vi "setUp.vi"(8 "error in (no error)":errorcluster, 11 "reference in":refnum<class "UnitTestIntClass.lvclass">) -> (0 "error out":errorcluster, 3 "reference in":refnum<class "UnitTestIntClass.lvclass">)   [LabVIEW 2011, in "UnitTestIntClass.lvclass"]
doc: "setUp runs prior to the test method during test execution. Use this method to initialize any object data required by your tests."
uses:
  UnitTestIntClass.lvclass
  UnitTestIntClass.lvclass/UnitTestIntClass.ctl
  IntClass/IntClass.lvclass
  <vilib>/addons/_JKI Toolkits/VI Tester/TestCase.llb/TestCase.lvclass
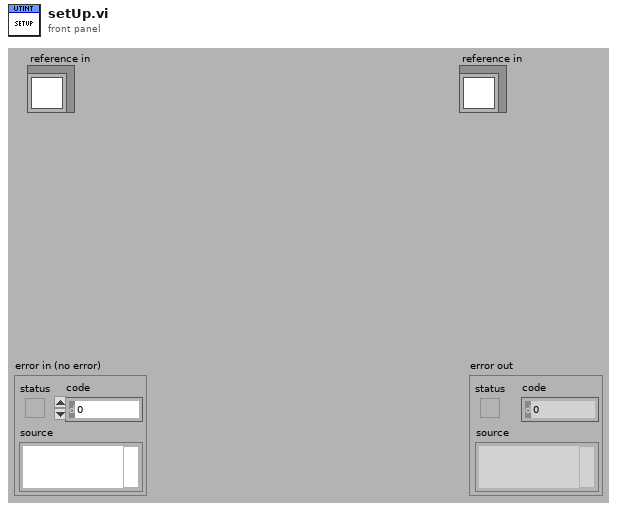
[diagram p1: front panel]
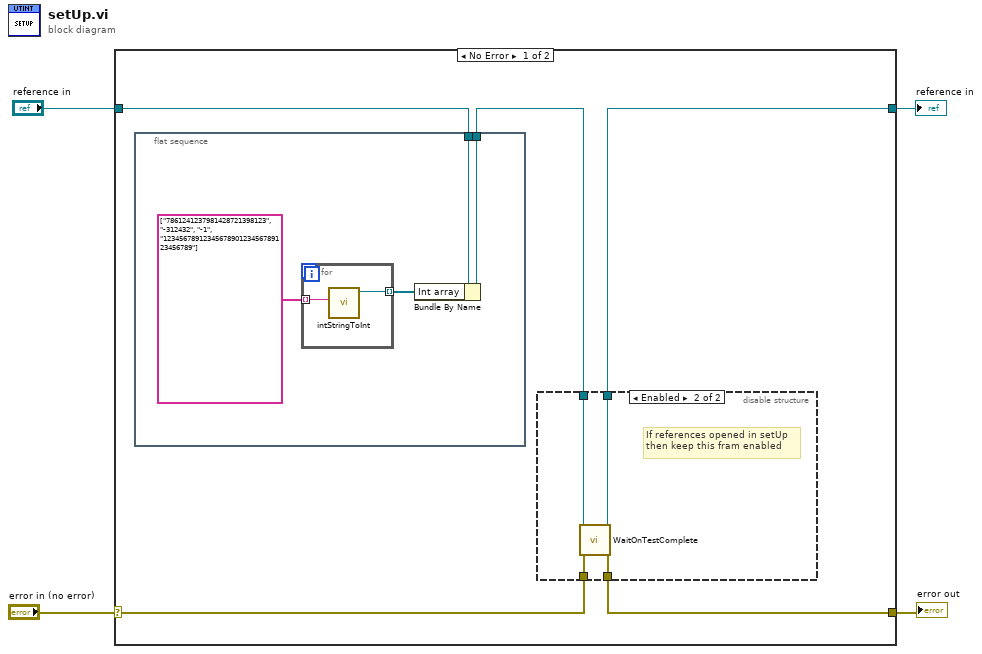
[diagram p0: block diagram]
diagram:
  n1 = case shown="No Error" "error in (no error)" {
    selector: "error in (no error)" -> [w6 w23]
    tunnel: [w5 w23] -> w3
    tunnel: [w7 w22] -> w1
    tunnel: "reference in" -> [w9 w22]
    frame No Error {
      n2 = flat-sequence {
        tunnel: w9 -> [w12]
        tunnel: [w11] -> w8
        frame #0 {
          n3 = for {
            tunnel: string[] ["7861241237981428721398123", "-312432", "-1", "1234567891234567890123456789123456789"] -> [w15] mode=indexing
            tunnel: [w14] -> w10 mode=indexing
            n4 = call "intStringToInt.vi"("String in"=w15) -> ("Int out"=w14:refnum<class "IntClass.lvclass">)  [unwired: 9 in, 1 out]
          }
          n5 = Bundle By Name(cluster=w12, "Int array"=w10) -> (w11:refnum<class "UnitTestIntClass.lvclass">)
        }
      }
      n6 = disable-structure shown="Enabled" {
        disable-tunnel: w8 -> [w17 w21]
        disable-tunnel: [w17 w20] -> w7
        disable-tunnel: w6 -> [w16 w19]
        disable-tunnel: [w16 w18] -> w5
        frame Disabled {
          # "If no references opened by\nsetUp then enable this frame"
        }
        frame Enabled {
          # "If references opened in setUp\nthen keep this fram enabled"
          n7 = call <vilib>:"WaitOnTestComplete.vi"("error in (no error)"=w19, "TestCase in"=w21) -> ("error out"=w18:errorcluster, "TestCase out"=w20:refnum<class "UnitTestIntClass.lvclass">)  [unwired: 8 in]
        }
      }
    }
    frame Error {
    }
  }
  "error out" <- w3
  "reference in" <- w1
